vi "FinBuild.vi"   [LabVIEW 2015]
uses:
  <vilib>/NXT/Block Support/NXT_InputPort.ctl
  <vilib>/NXT/Block Support/NXT_OutputPort.ctl
  <vilib>/NXT/Dual Mode Library/Sensors/Light_On.vi
  <vilib>/NXT/Dual Mode Library/Sensors/Sonar_cm.vi
  <vilib>/NXT/NXTIO Xnodes/NXTIONodeSubVIs/NXTMoveMotors.vi
  <vilib>/NXT/Dual Mode Library/Waits/Wait_Num(msec).vi
  <vilib>/NXT/Subs/LVHSConnector.ctl
  <vilib>/NXT/NXTIO Xnodes/AddressXNode/NXTIOAddress.xnode
  <vilib>/NXT/NXTIO Xnodes/NXTIOXNode/NXTIO.xnode
  <vilib>/NXT/LegoClasses/BrickReference/BrickReference.lvclass
types:
  T1 = typedef "NXT_OutputPort.ctl" = u8
  T2 = typedef "NXT_InputPort.ctl" = u32
  T3 = typedef "LVHSConnector.ctl" = refnum<class "BrickReference.lvclass">
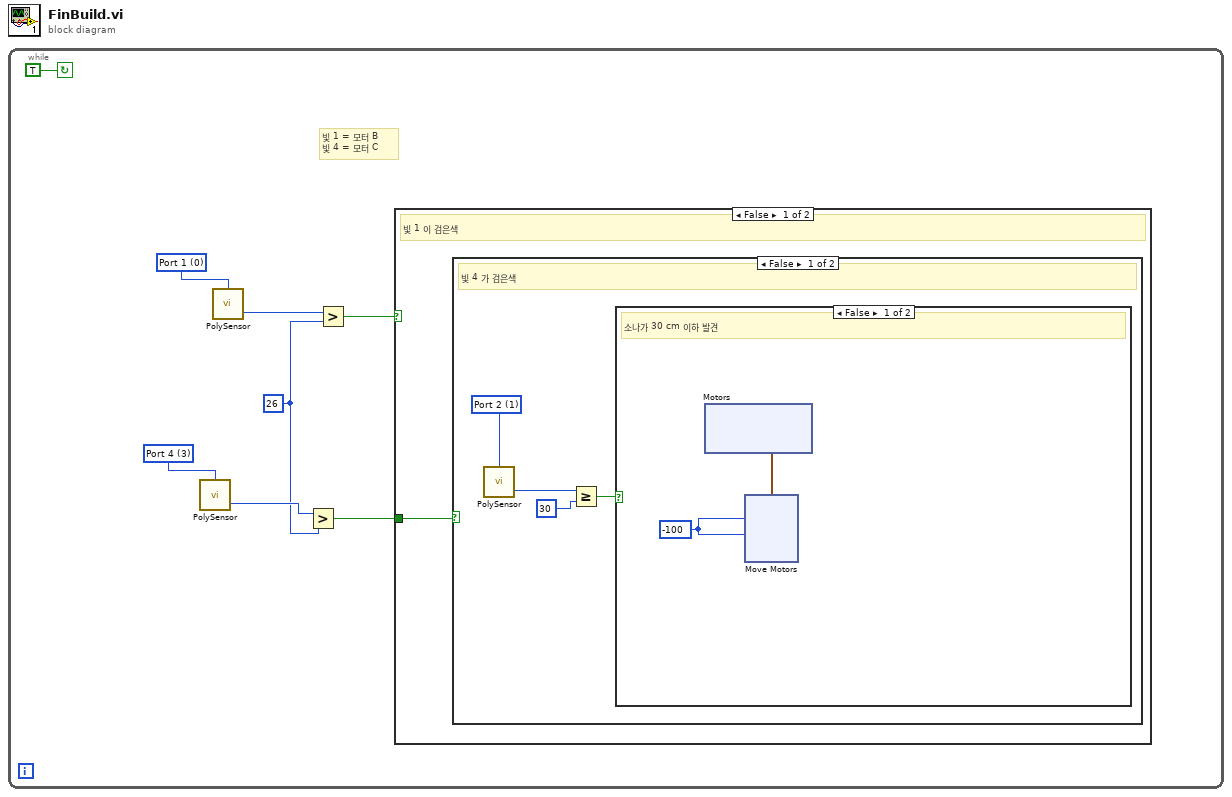
[diagram p0: block diagram]
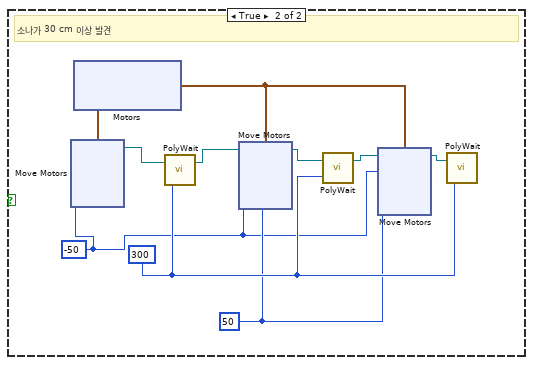
[diagram p2: hidden frame]
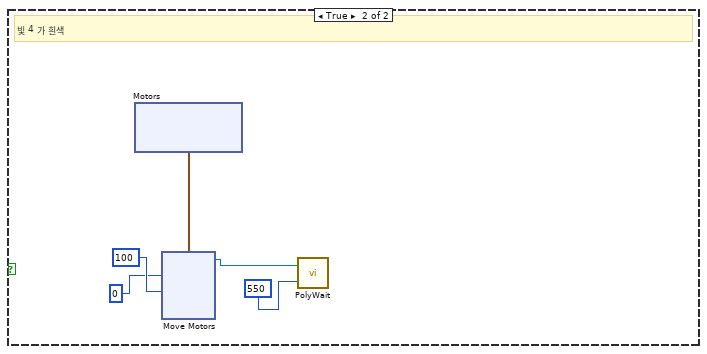
[diagram p3: hidden frame]
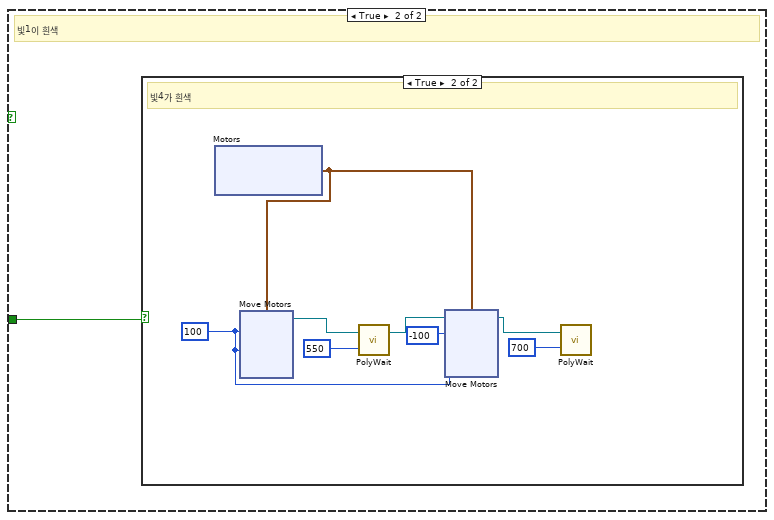
[diagram p4: hidden frame]
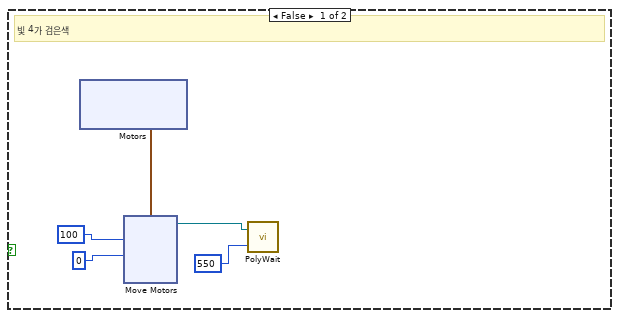
[diagram p5: hidden frame]
diagram:
  n1 = while {
    stop <- TRUE continue-if-true
    w1 = i16 26 ("y")
    w6 = T2 0 items=["Port 1", "Port 2", "Port 3", "Port 4"] ("Port (Port 3)")
    w5 = T2 3 items=["Port 1", "Port 2", "Port 3", "Port 4"] ("Port (Port 3)")
    # "빛 1 = 모터 B\n빛 4 = 모터 C"
    n2 = call-poly <vilib>:"PolySensor.vi"("Port (Port 3)"=w5) -> ("Scaled Value"=w7:i16)  [unwired: 2 in, 1 out]
    n3 = call-poly <vilib>:"PolySensor.vi"("Port (Port 3)"=w6) -> ("Scaled Value"=w8:i16)  [unwired: 2 in, 1 out]
    n4 = Greater?(x=w7, y=w1) -> (0:w3:bool)
    n5 = Greater?(x=w8, y=w1) -> (0:w4:bool)
    n6 = case shown="False" w4 {
      tunnel: w3 -> [w9 w73]
      frame False {
        # "빛 1 이 검은색"
        n7 = case shown="False" w9 {
          frame False {
            w10 = T2 1 items=["Port 1", "Port 2", "Port 3", "Port 4"] ("Port (Port 4)")
            # "빛 4 가 검은색"
            n8 = call-poly <vilib>:"PolySensor.vi"("Port (Port 4)"=w10) -> ("Distance (cm)"=w13:i16)  [unwired: 2 in, 1 out]
            n9 = Greater Or Equal?(x=w13, y=i16 30) -> (x >= y?=w11:bool)
            n10 = case shown="False" w11 {
              frame False {
                w14 = i16 -100 ("y")
                # "소나가 30 cm 이하 발견"
                n11 = xnode "Motors"() -> ("Motor"=w15:cluster{"Port":T1, "Port":T1})
                n12 = xnode "Move Motors"("Power/Speed 2"=w14, "Power/Speed 1"=w14, "Motors"=w15) -> ()  [unwired: 1 in, 1 out]
              }
              frame True {
                w32 = i16 300 ("y")
                w31 = i16 50 ("y")
                w30 = i16 -50 ("y")
                # "소나가 30 cm 이상 발견"
                n13 = xnode "Motors"() -> ("Motor"=w33:cluster{"Port":T1, "Port":T1})
                n14 = xnode "Move Motors"("Power/Speed 2"=w30, "Power/Speed 1"=w30, "Motors"=w33) -> ("NXT/EV3"=w29:T3)  [unwired: 1 in]
                n15 = call-poly <vilib>:"PolyWait.vi"("Time (100 msec)"=w32, "NXT/EV3"=w29) -> ("NXT/EV3"=w28:T3)  [unwired: 2 in]
                n16 = xnode "Move Motors"("Power/Speed 2"=w30, "Power/Speed 1"=w31, "Motors"=w33, "NXT/EV3"=w28) -> ("NXT/EV3"=w27:T3)
                n17 = call-poly <vilib>:"PolyWait.vi"("Time (100 msec)"=w32, "NXT/EV3"=w27) -> ("NXT/EV3"=w26:T3)  [unwired: 2 in]
                n18 = xnode "Move Motors"("Power/Speed 2"=w31, "Power/Speed 1"=w30, "Motors"=w33, "NXT/EV3"=w26) -> ("NXT/EV3"=w25:T3)
                n19 = call-poly <vilib>:"PolyWait.vi"("Time (100 msec)"=w32, "NXT/EV3"=w25) -> ()  [unwired: 2 in, 1 out]
              }
            }
          }
          frame True {
            # "빛 4 가 흰색"
            n20 = xnode "Motors"() -> ("Motor"=w63:cluster{"Port":T1, "Port":T1})
            n21 = xnode "Move Motors"("Power/Speed 2"=i16 100 ("y"), "Power/Speed 1"=i16 0 ("y"), "Motors"=w63) -> ("NXT/EV3"=w61:T3)  [unwired: 1 in]
            n22 = call-poly <vilib>:"PolyWait.vi"("Time (100 msec)"=i16 550 ("y"), "NXT/EV3"=w61) -> ()  [unwired: 2 in, 1 out]
          }
        }
      }
      frame True {
        # "빛1이 흰색"
        n23 = case shown="True" w73 {
          frame False {
            # "빛 4가 검은색"
            n24 = xnode "Motors"() -> ("Motor"=w78:cluster{"Port":T1, "Port":T1})
            n25 = xnode "Move Motors"("Power/Speed 2"=i16 0 ("y"), "Power/Speed 1"=i16 100 ("y"), "Motors"=w78) -> ("NXT/EV3"=w76:T3)  [unwired: 1 in]
            n26 = call-poly <vilib>:"PolyWait.vi"("Time (100 msec)"=i16 550 ("y"), "NXT/EV3"=w76) -> ()  [unwired: 2 in, 1 out]
          }
          frame True {
            w88 = i16 100 ("y")
            # "빛4가 흰색"
            n27 = xnode "Motors"() -> ("Motor"=w95:cluster{"Port":T1, "Port":T1})
            n28 = xnode "Move Motors"("Power/Speed 2"=w88, "Power/Speed 1"=w88, "Motors"=w95) -> ("NXT/EV3"=w94:T3)  [unwired: 1 in]
            n29 = call-poly <vilib>:"PolyWait.vi"("Time (100 msec)"=i16 550 ("y"), "NXT/EV3"=w94) -> ("NXT/EV3"=w93:T3)  [unwired: 2 in]
            n30 = xnode "Move Motors"("Power/Speed 2"=w88, "Power/Speed 1"=i16 -100 ("y"), "Motors"=w95, "NXT/EV3"=w93) -> ("NXT/EV3"=w92:T3)
            n31 = call-poly <vilib>:"PolyWait.vi"("Time (100 msec)"=i16 700 ("y"), "NXT/EV3"=w92) -> ()  [unwired: 2 in, 1 out]
          }
        }
      }
    }
  }
